vi "KB-CalCorssPoint.vi"(6 "R":dbl caption="r", 8 "b":dbl, 9 "a":dbl, 10 "X":dbl[](array[numeric]), 11 "Y":dbl[](array[numeric])) -> (1 "b1":dbl, 2 "k1":dbl, 3 "X1Y1X2Y2":cluster{"x1":dbl, "y1":dbl, "x2":dbl, "y2":dbl})   [LabVIEW 2015]
uses:
  <vilib>/Analysis/NI_AALPro.lvlib
panel:
  out "y2":dbl
  out "x2":dbl
  out "y1":dbl
  out "x1":dbl
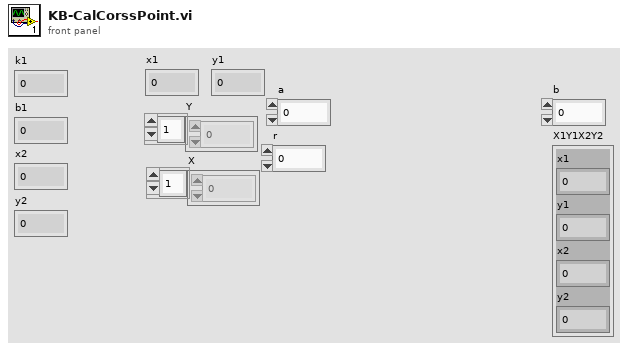
[diagram p1: front panel]
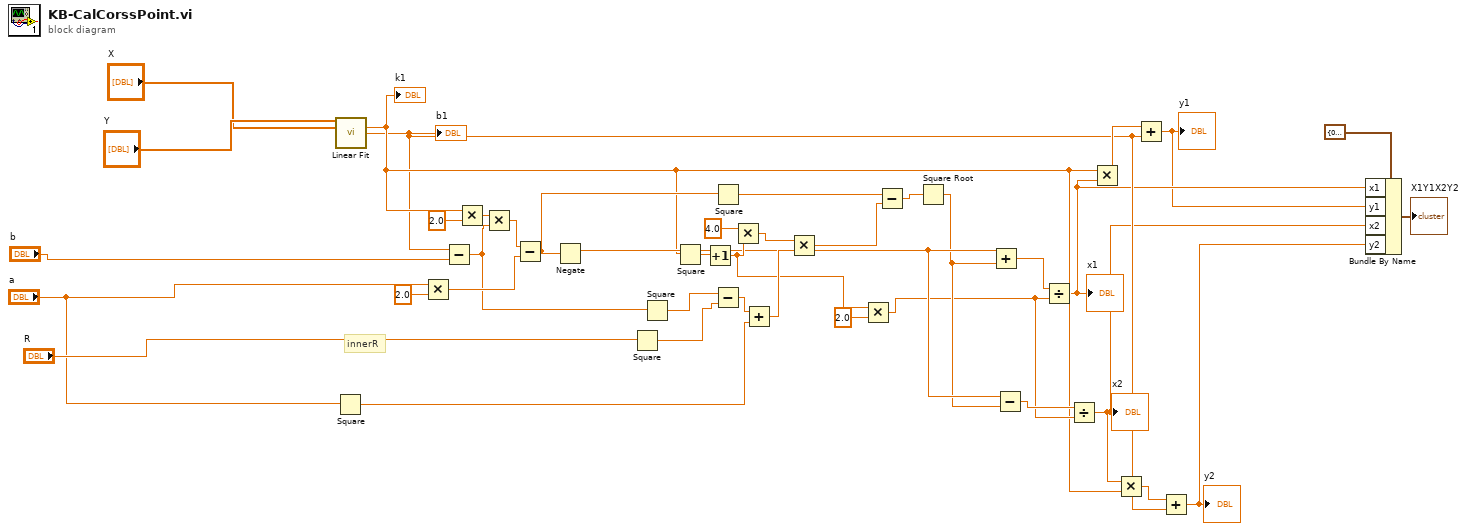
[diagram p0: block diagram]
diagram:
  # "innerR"
  n1 = Square(x="a") -> (x^2=w26:dbl)
  n2 = call <vilib>:"Linear Fit.vi"("Y"="Y", "X"="X") -> ("slope"=w14:dbl, "intercept"=w12:dbl)  [unwired: 9 in, 3 out]
  "k1" <- w14
  "b1" <- w12
  n3 = Multiply(x="a", y=2.0) -> (x*y=w36:dbl)
  n4 = Subtract(x=w12, y="b") -> (x-y=w31:dbl)
  n5 = Multiply(x=w14, y=2.0) -> (x*y=w39:dbl)
  n6 = Multiply(x=w39, y=w31) -> (x*y=w38:dbl)
  n7 = Subtract(x=w38, y=w36) -> (x-y=w35:dbl)
  n8 = Negate(x=w35) -> (-x=w18:dbl)
  n9 = Square(x="R") -> (x^2=w28:dbl)
  n10 = Square(x=w31) -> (x^2=w29:dbl)
  n11 = Square(x=w14) -> (x^2=w32:dbl)
  n12 = Increment(x=w32) -> (x+1=w21:dbl)
  n13 = Square(x=w35) -> (x^2=w34:dbl)
  n14 = Subtract(x=w29, y=w28) -> (x-y=w27:dbl)
  n15 = Multiply(x=4.0, y=w21) -> (x*y=w30:dbl)
  n16 = Add(x=w27, y=w26) -> (x+y=w25:dbl)
  n17 = Multiply(x=w30, y=w25) -> (x*y=w24:dbl)
  n18 = Multiply(x=w21, y=2.0) -> (x*y=w15:dbl)
  n19 = Subtract(x=w34, y=w24) -> (x-y=w23:dbl)
  n20 = Square Root(x=w23) -> (sqrt(x)=w17:dbl)
  n21 = Add(x=w18, y=w17) -> (x+y=w22:dbl)
  n22 = Subtract(x=w18, y=w17) -> (x-y=w16:dbl)
  n23 = Divide(x=w22, y=w15) -> (x/y=w5:dbl)
  "x1" <- w5
  n24 = Divide(x=w16, y=w15) -> (x/y=w3:dbl)
  "x2" <- w3
  n25 = Multiply(x=w14, y=w5) -> (x*y=w19:dbl)
  n26 = Multiply(x=w3, y=w14) -> (x*y=w13:dbl)
  n27 = Add(x=w19, y=w12) -> (x+y=w4:dbl)
  "y1" <- w4
  n28 = Add(x=w13, y=w12) -> (x+y=w2:dbl)
  "y2" <- w2
  n29 = Bundle By Name(cluster=cluster{"x1":dbl, "y1":dbl, "x2":dbl, "y2":dbl} {"x1"=0.0, "y1"=0.0, "x2"=0.0, "y2"=0.0}, "x1"=w5, "y1"=w4, "x2"=w3, "y2"=w2) -> (→"X1Y1X2Y2":cluster{"x1":dbl, "y1":dbl, "x2":dbl, "y2":dbl})
